vi "Rebuild from Tree.vi"(8 "error in (no error)":errorcluster, 10 "Tag":string, 11 "Tree Manager in":refnum<class "Tree Manager.lvclass">) -> (0 "error out":errorcluster, 2 "Rebuilt Item":refnum<class "Data Item.lvclass">, 3 "Tree Manager out":refnum<class "Tree Manager.lvclass">)   [LabVIEW 2023, in "VILab.lvlib" / "Tree Manager.lvclass"]
uses:
  Tree Manager.lvclass
  Data Item.lvclass
  Tree Manager.lvclass/Tree Manager.ctl
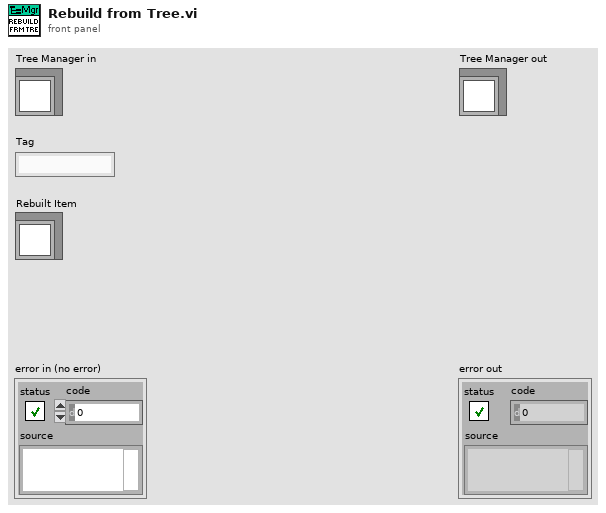
[diagram p1: front panel]
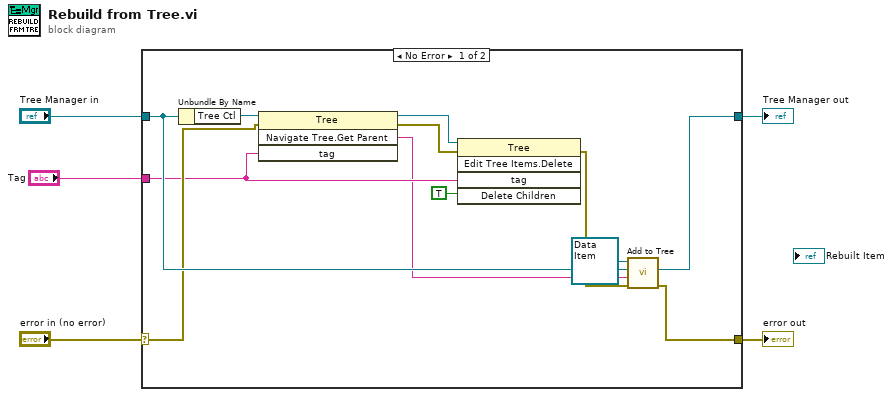
[diagram p0: block diagram]
diagram:
  n1 = case shown="No Error" "error in (no error)" {
    selector: "error in (no error)" -> [w13 w19]
    tunnel: [w7 w19] -> w4
    tunnel: [w8 w18] -> w2
    tunnel: "Tree Manager in" -> [w16 w18]
    tunnel: "Tag" -> [w12 _]
    frame No Error {
      n2 = Unbundle By Name(w16) -> ("Tree Ctl"=w14:refnum<vi>)
      n3 = invoke class="Tree" method="Navigate Tree.Get Parent"(reference=w14, error in=w13, "tag"=w12) -> (reference out=w11:refnum<vi>, error out=w10:errorcluster, "Navigate Tree:Get Parent"=w9:string)  [unwired: 1 in, 1 out]
      n4 = invoke on="Delete" class="Tree" method="Edit Tree Items.Delete"(reference=w11, error in=w10, "tag"=w12, "Delete Children"=TRUE ("Delete Children?")) -> (error out=w15:errorcluster)  [unwired: 1 in, 4 out]
      n5 = call-dynamic "Add to Tree.vi"("error in (no error)"=w15, "Parent Tag"=w9, "Tree Manager in"=w16, "Data Item in"=refnum<class "Data Item.lvclass"> refnum) -> ("error out"=w7:errorcluster, "Tree Manager out"=w8:refnum<class "Tree Manager.lvclass">)  [unwired: 5 in, 1 out]
    }
    frame Error {
    }
  }
  "error out" <- w4
  "Tree Manager out" <- w2
